vi "2D Real FFT.vi"(8 "n":i32=-1, 9 "m":i32=-1, 10 "shift?":bool, 11 "X":dbl[][](array[numeric])) -> (0 "error":i32, 3 "FFT {X}":cdb[][](array[numeric]))   [LabVIEW 2010, in "NI_AALPro.lvlib"]
doc: "Computes the fast Fourier transform (FFT) of the input sequence <B>X</B>. Wire data to the <B>X</B> input to determine the polymorphic instance to use or manually select the instance."
uses:
  NI_AALPro.lvlib
  lvanlys.dll
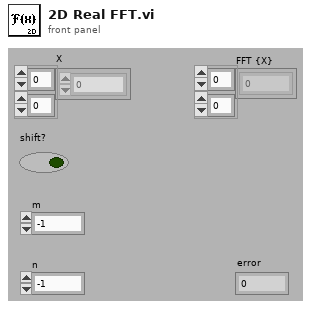
[diagram p1: front panel]
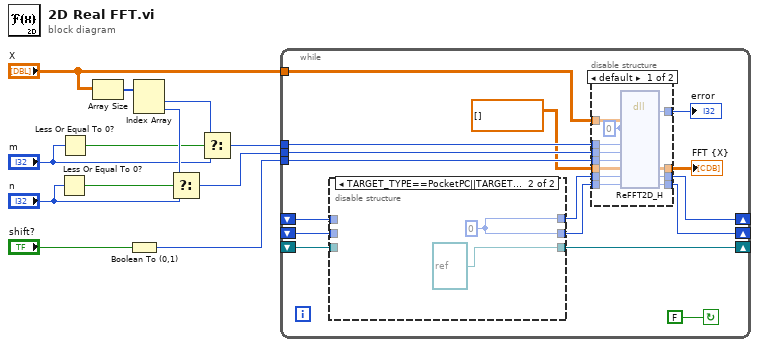
[diagram p0: block diagram]
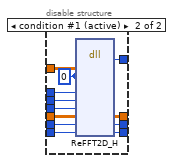
[diagram p2: hidden frame]
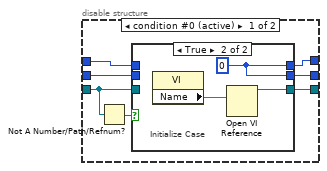
[diagram p3: hidden frame]
diagram:
  n1 = Less Or Equal To 0?(x="n") -> (x <= 0?=w3:bool)
  n2 = Less Or Equal To 0?(x="m") -> (x <= 0?=w4:bool)
  n3 = Array Size(array="X") -> (size(s)=w11:i32[])
  n4 = Boolean To (0,1)(Boolean="shift?") -> (0, 1=w1:i16)
  n5 = Index Array(array=w11) -> (element #1=w10:i32, element #2=w9:i32)  [unwired: 2 in]
  n6 = Select(t=w9, s=w3, f="n") -> (s? t:f=w7:i32)
  n7 = Select(t=w10, s=w4, f="m") -> (s? t:f=w8:i32)
  n8 = while {
    shift-left: _ -> [w26]
    shift-right: [w21] -> _
    tunnel: "X" -> [w27]
    shift-right: [w25] -> _
    shift-left: _ -> [w24]
    shift-right: [w20] -> _
    shift-left: _ -> [w19]
    tunnel: w8 -> [w18]
    tunnel: w7 -> [w17]
    tunnel: w1 -> [w16]
    stop <- FALSE continue-if-true
    n9 = disable-structure shown="TARGET_TYPE==PocketPC||TARGET_TYPE==PalmOS||TARGET_TYPE==FPGA||TARGET_TYPE==Embedded" {
      disable-tunnel: w24 -> [w57 _]
      disable-tunnel: [w58 refnum<vi> refnum ("VI Refnum")] -> w25
      disable-tunnel: w26 -> [w56 _]
      disable-tunnel: [w55 w67] -> w23
      disable-tunnel: [w54 w67] -> w22
      disable-tunnel: w19 -> [w53 _]
      frame condition #0 (active) {
        n10 = Not A Number/Path/Refnum?(number/path/refnum=w57) -> (NaN/Path/Refnum?=w59:bool)
        n11 = case shown="True" w59 {
          tunnel: [w62 w64] -> w58
          tunnel: w57 -> [w62 _]
          tunnel: w56 -> [w61 _]
          tunnel: [w61 w65] -> w55
          tunnel: [w60 w65] -> w54
          tunnel: w53 -> [w60 _]
          frame False {
          }
          frame True {
            w65 = 0 ("error")
            # "Initialize Case"
            n12 = property class="VI"() -> ("Name"=w63:string)  [unwired: 2 in, 2 out]
            n13 = Open VI Reference(vi path=w63) -> (vi reference=w64:refnum<vi>)  [unwired: 5 in, 1 out]
          }
        }
      }
      frame condition #1 {
        w67 = 0 ("t")
      }
    }
    n14 = disable-structure shown="default" {
      disable-tunnel: w27 -> [w40 w52]
      disable-tunnel: w23 -> [w39 w51]
      disable-tunnel: w22 -> [w38 w50]
      disable-tunnel: [w37 w49] -> w21
      disable-tunnel: [w36 w48] -> w20
      disable-tunnel: w18 -> [w35 w47]
      disable-tunnel: w17 -> [w34 w46]
      disable-tunnel: w16 -> [w33 w45]
      disable-tunnel: [w32 w44] -> w14
      disable-tunnel: [w31 w43] -> w15
      disable-tunnel: cdb[][] [] ("FFT {X}") -> [w29 w41]
      frame condition #0 {
        w30 = 0 ("orgRow")
        n15 = dll-call lib="C:/Program Files/National Instruments/LabVIEW 2010/resource/lvanlys.dll" fn="ReFFT2D_H"("X"=w40, "orgRow"=w30, "orgCol"=w30, "rowsFFT"=w35, "colsFFT"=w34, "shift"=w33, w29, "tblRow"=w39, "tblCol"=w38) -> (w31:i32, w32:cdb[][], "tblRow"=w37:i32, "tblCol"=w36:i32)  [unwired: 9 in, 2 out]
      }
      frame condition #1 (active) {
        w42 = 0 ("orgRow")
        n16 = dll-call lib="C:/Program Files/National Instruments/LabVIEW 2010/resource/lvanlys.dll" fn="ReFFT2D_H"("xH"=w52, "orgRow"=w42, "orgCol"=w42, "rowsFFT"=w47, "colsFFT"=w46, "shift"=w45, "yH"=w41, "tblRow"=w51, "tblCol"=w50) -> ("return type"=w43:i32, "yH"=w44:cdb[][], "tblRow"=w49:i64, "tblCol"=w48:i64)  [unwired: 9 in, 2 out]
      }
    }
    "FFT {X}" <- w14
    "error" <- w15
  }
